vi "Traverse-Move-Low.vi"(8 "error in":errorcluster, 9 "Trav Command":T1 items=["Set Reference", "Read Position", "Move", "StopMotors"], 10 "Settings":T3, 11 "Position Info IN":T2) -> (0 "error out":errorcluster, 3 "Position Info OUT":T2)   [LabVIEW 2017]
uses:
  TypeDefs/Position-Info-TD.ctl
  Settings/Settings-Control.ctl
  TypeDefs/Trav-Command-TD.ctl
  <userlib>/ICNC/ICNC2.lvlib
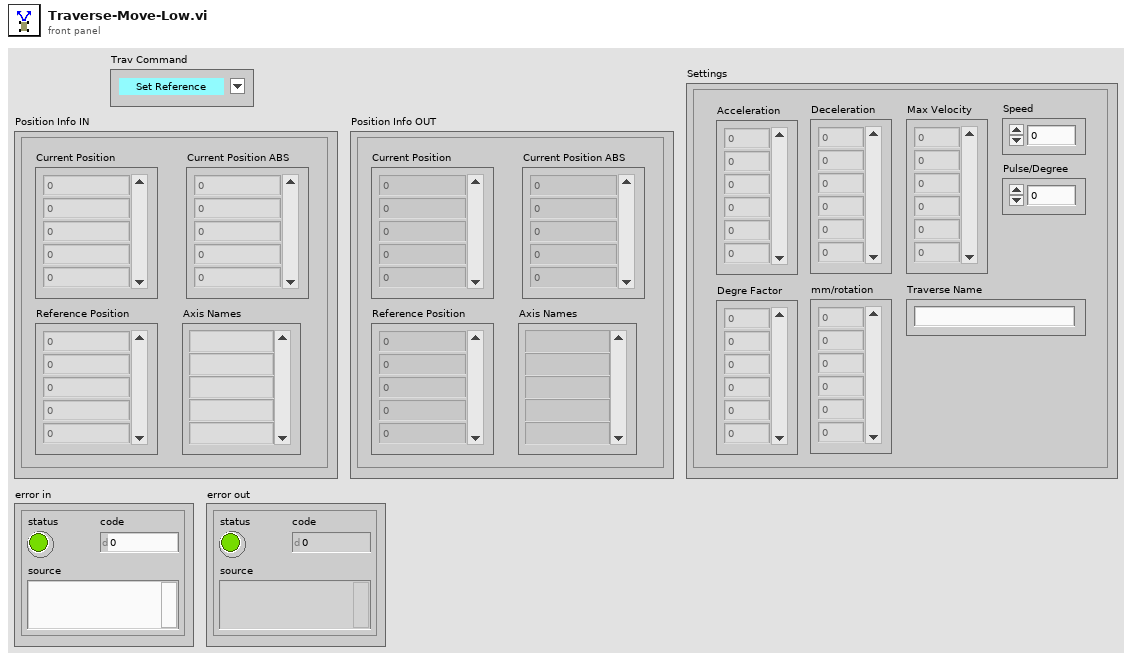
[diagram p1: front panel]
types:
  T1 = typedef "Trav-Command-TD.ctl" = u16
  T2 = typedef "Position-Info-TD.ctl" = cluster{"Current Position ABS":dbl[], "Current Position":dbl[], "Reference Position":dbl[], "Axis Names":string[]}
  T3 = typedef "Settings-Control.ctl" = cluster{"Acceleration":dbl[], "Deceleration":dbl[], "Max Velocity":dbl[], "Speed":dbl, "Pulse/Degree":dbl, "Degre Factor":dbl[], "mm/rotation":dbl[], "Traverse Name":string}
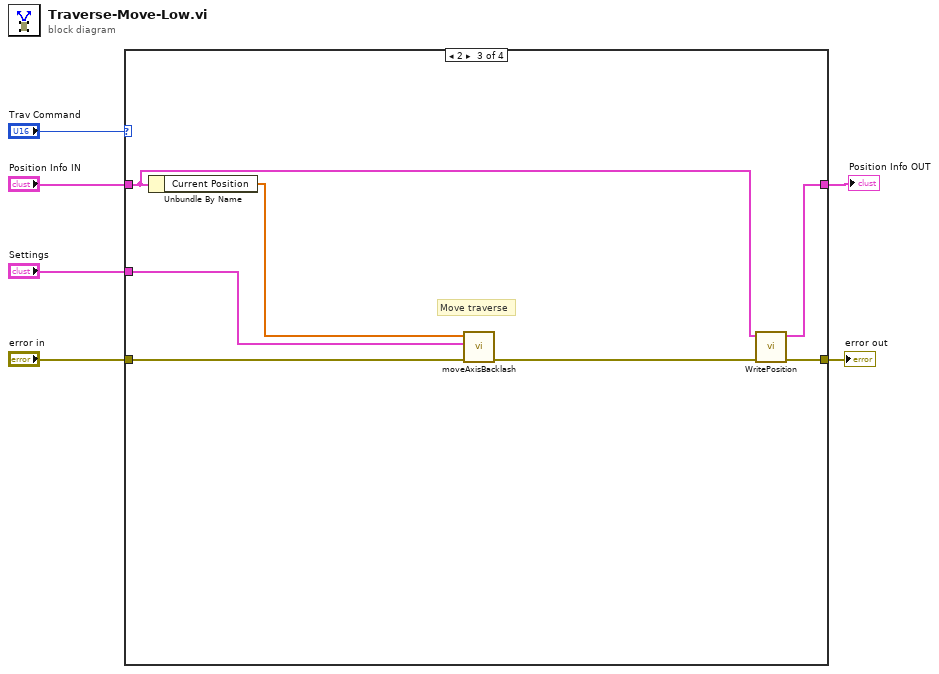
[diagram p0: block diagram]
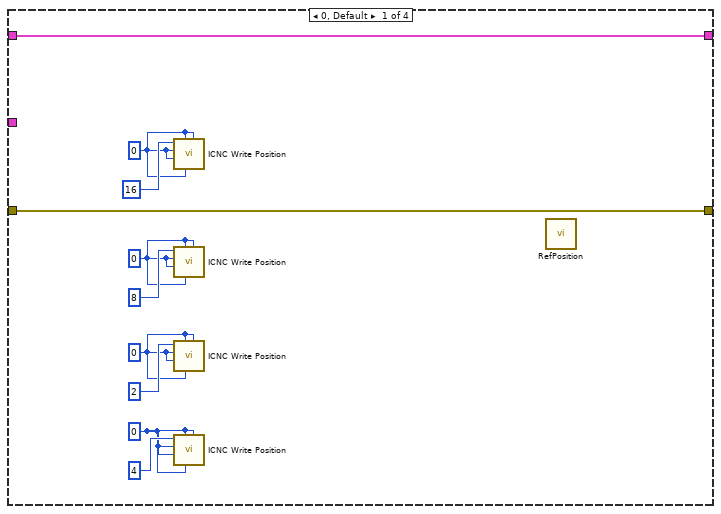
[diagram p2: hidden frame]
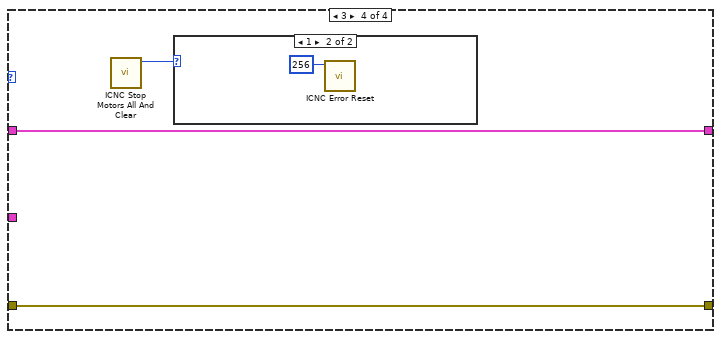
[diagram p4: hidden frame]
diagram:
  n1 = case shown="2" "Trav Command" {
    tunnel: "Position Info IN" -> [w16 w18 w21 w27]
    tunnel: [w16 w18 w20 w27] -> w4
    tunnel: "Settings" -> [_ _ w24 _]
    tunnel: [w7 w17 w25 w26] -> w2
    tunnel: "error in" -> [w7 w17 w23 w26]
    frame 0, Default {
      w9 = 0
      w8 = 0
      w12 = 0
      w14 = 0
      n2 = call <userlib>:"ICNC Write Position.vi"("PositionB"=w9, "PositionA"=w9, "PositionZ"=w9, "PositionY"=w9, "PositionX"=w9, "Axis"=16) -> ()  [unwired: 4 in, 2 out]
      n3 = call <userlib>:"ICNC Write Position.vi"("PositionB"=w8, "PositionA"=w8, "PositionZ"=w8, "PositionY"=w8, "PositionX"=w8, "Axis"=8) -> ()  [unwired: 4 in, 2 out]
      n4 = call <userlib>:"ICNC Write Position.vi"("PositionB"=w14, "PositionA"=w14, "PositionZ"=w14, "PositionY"=w14, "PositionX"=w14, "Axis"=2) -> ()  [unwired: 4 in, 2 out]
      n5 = call <userlib>:"ICNC Write Position.vi"("PositionB"=w12, "PositionA"=w12, "PositionZ"=w12, "PositionY"=w12, "PositionX"=w12, "Axis"=4) -> ()  [unwired: 4 in, 2 out]
      n6 = call "RefPosition.vi"() -> ()  [unwired: 10 in]
    }
    frame 1 {
      # "read position info from file"
    }
    frame 2 {
      # "Move traverse"
      n7 = Unbundle By Name(w21) -> ("Current Position"=w19:dbl[])
      n8 = call "moveAxisBacklash.vi"("error in (no error)"=w23, "Settings"=w24, "Current Position"=w19) -> ("error out"=w22:errorcluster)  [unwired: 8 in]
      n9 = call "WritePosition.vi"("error in"=w22, "Position Info"=w21) -> ("error out"=w25:errorcluster, "Position Info"=w20:T2)  [unwired: 8 in]
    }
    frame 3 {
      n10 = call <userlib>:"ICNC Stop Motors All And Clear.vi"() -> ("function return"=w28:u32)  [unwired: 10 in, 1 out]
      n11 = case shown="1" w28 {
        frame 0, Default {
        }
        frame 1 {
          n12 = call <userlib>:"ICNC Error Reset.vi"("ErrorBits"=256) -> ()  [unwired: 9 in, 2 out]
        }
      }
    }
  }
  "error out" <- w2
  "Position Info OUT" <- w4
